vi "Factorial.vi"() -> ()   [LabVIEW 2024]
panel:
  out "Numeric 2":dbl
  in  "Numeric":dbl
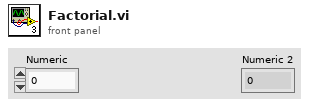
[diagram p1: front panel]
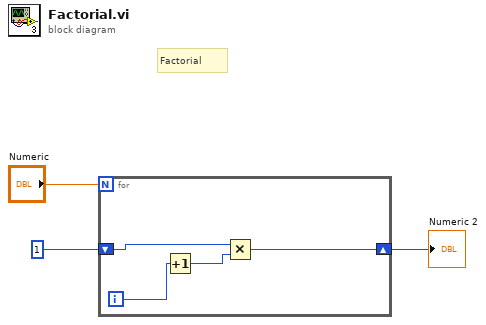
[diagram p0: block diagram]
diagram:
  # "Factorial"
  n1 = for {
    N: "Numeric" -> [_]
    shift-right: [w5] -> w2
    shift-left: 1 -> [w4]
    i -> [w7]
    n2 = Increment(x=w7) -> (x+1=w6:i32)
    n3 = Multiply(x=w4, y=w6) -> (x*y=w5:i32)
  }
  "Numeric 2" <- w2
